vi "CoMP-S Mechanism - AISAS Motor Controller - MK.vi"(8 "Steps/sec (3-365)":dbl=15.0, 9 "Steps":dbl=10.0, 10 "Motor Direction":T1=enum."Rotation Counter Clockwise", 11 "Motor":T2=enum."Rotation") -> (0 "Read Buffer Out":string="\n", 1 "Bytes Read":u32=1, 2 "Estimated time [sec]":dbl=0.9876666666666667, 3 "sec":ext=0.62100000000000000003)   [LabVIEW 2014]
doc: "Rotation Definition when Looking at the Sun. CCW, Right is CW, Optimum speed is 10 steps/s\n\nDiffuser opens with 1200 total steps, optimum speed is 10 steps/s\n\nObjective Lens\n\n\nvelocity = 730,88/steps.p.sec"
uses:
  AISAS Mechanism Action Type Def.ctl
  AISAS Mechanism Action Direction Type Def.ctl
panel:
  out "ERROR":bool
  in  "bytes  to read":i32=1
  # "Time [sec]"
  # "k"
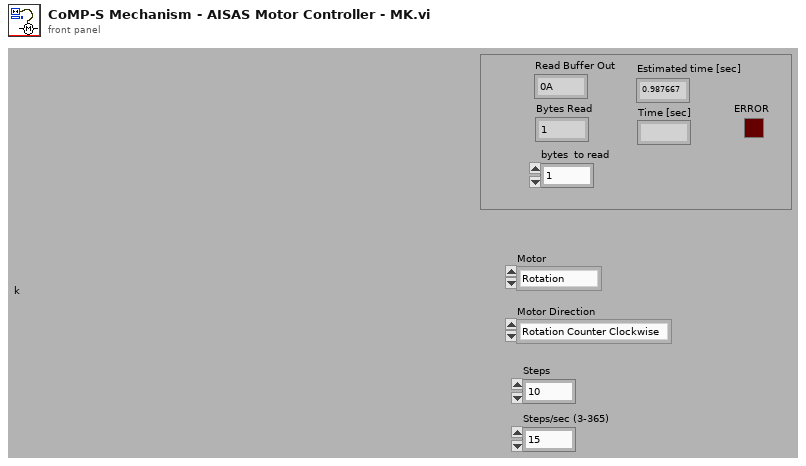
[diagram p1: front panel]
types:
  T1 = typedef "AISAS Mechanism Action Direction Type Def.ctl" = enum16{"Diffuser Closed", "Diffuser Open", "Objective Lens Away", "Objective Lens Closer", "Rotation Counter Clockwise", "Rotation Clockwise"}
  T2 = typedef "AISAS Mechanism Action Type Def.ctl" = enum16{"Diffuser", "Objective Lens", "Rotation"}
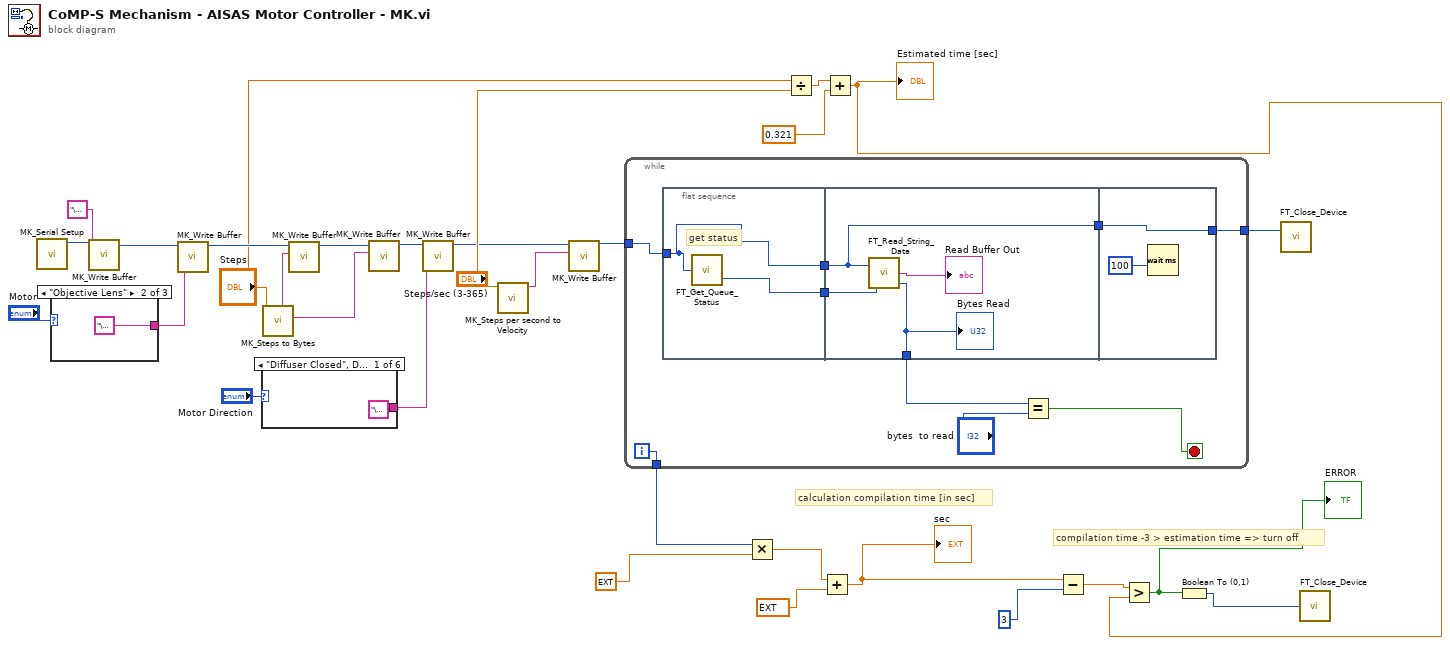
[diagram p0: block diagram]
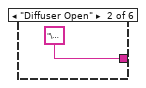
[diagram p2: hidden frame]
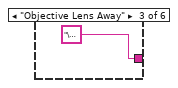
[diagram p3: hidden frame]
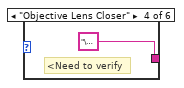
[diagram p4: hidden frame]
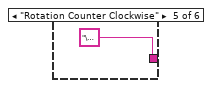
[diagram p5: hidden frame]
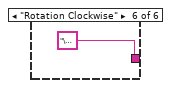
[diagram p6: hidden frame]
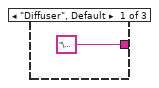
[diagram p7: hidden frame]
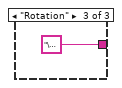
[diagram p8: hidden frame]
diagram:
  # "compilation time -3 > estimation time => turn off"
  # "calculation compilation time [in sec]"
  n1 = call "MK_Serial Setup.vi"() -> ("Handle"=w17:u32)  [unwired: 11 in]
  n2 = case shown="\"Objective Lens\"" "Motor" {
    tunnel: ["\u0003" "\u0004" "\u0002"] -> w14
    frame "Diffuser", Default {
    }
    frame "Objective Lens" {
    }
    frame "Rotation" {
    }
  }
  n3 = call "MK_Write Buffer.vi"("Buffer"="\u0001", "Handle in"=w17) -> ("Handle out"=w13:u32)  [unwired: 9 in]
  n4 = call "MK_Write Buffer.vi"("Buffer"=w14, "Handle in"=w13) -> ("Handle out"=w9:u32)  [unwired: 9 in]
  n5 = case shown="\"Diffuser Closed\", Default" "Motor Direction" {
    tunnel: ["\u0000" "\u0001" "\u0000" "\u0001" "\u0001" "\u0000"] -> w6
    frame "Diffuser Closed", Default {
    }
    frame "Diffuser Open" {
    }
    frame "Objective Lens Away" {
    }
    frame "Objective Lens Closer" {
      # "<Need to verify"
    }
    frame "Rotation Counter Clockwise" {
    }
    frame "Rotation Clockwise" {
    }
  }
  n6 = call "MK_Steps to Bytes.vi"("Steps"="Steps") -> ("Hi Byte"=w10:string, "Lo Byte"=w12:string)  [unwired: 9 in]
  n7 = call "MK_Write Buffer.vi"("Buffer"=w12, "Handle in"=w9) -> ("Handle out"=w11:u32)  [unwired: 9 in]
  n8 = call "MK_Write Buffer.vi"("Buffer"=w10, "Handle in"=w11) -> ("Handle out"=w5:u32)  [unwired: 9 in]
  n9 = call "MK_Write Buffer.vi"("Buffer"=w6, "Handle in"=w5) -> ("Handle out"=w3:u32)  [unwired: 9 in]
  n10 = call "MK_Steps per second to Velocity.vi"("Steps/sec (3-365)"="Steps/sec (3-365)") -> ("Velocity"=w2:string)  [unwired: 10 in]
  n11 = call "MK_Write Buffer.vi"("Buffer"=w2, "Handle in"=w3) -> ("Handle out"=w1:u32)  [unwired: 9 in]
  n12 = while {
    tunnel: w1 -> [w48]
    tunnel: [w42] -> w28
    tunnel: [w40] -> w30
    i -> [w42]
    stop <- w43 stop-if-true
    n13 = flat-sequence {
      tunnel: w48 -> [w49]
      tunnel: [w50] -> w47
      tunnel: [w49] -> w46
      tunnel: w47 -> [w54]
      tunnel: w46 -> [w51]
      tunnel: [w52] -> w44
      tunnel: [w51] -> w41
      tunnel: w41 -> [w55]
      tunnel: [w55] -> w40
      frame #0 {
        # "get status"
        n14 = call "FT_Get_Queue_Status.vi"("Handle"=w49) -> ("Bytes Waiting"=w50:u32)  [unwired: 1 out]
      }
      frame #1 {
        n15 = call "FT_Read_String_Data.vi"("Handle"=w51, "Bytes To Read"=w54) -> ("Read Data"=→"Read Buffer Out":string, "Bytes Read"=w52:u32)  [unwired: 1 out]
        "Bytes Read" <- w52
      }
      frame #2 {
        n16 = Wait (ms)(milliseconds to wait=u32 100) -> ()  [unwired: 1 out]
      }
    }
    n17 = Equal?(x=w44, y="bytes  to read") -> (x = y?=w43:bool)
  }
  n18 = Multiply(x=w28, y=ext 0.1) -> (x*y=w26:ext)
  n19 = Divide(x="Steps", y="Steps/sec (3-365)") -> (x/y=w25:dbl)
  n20 = Add(x=w26, y=ext 0.32099999999999999999) -> (x+y=w23:ext)
  "sec" <- w23
  n21 = Add(x=w25, y=0.321) -> (x+y=w20:dbl)
  "Estimated time [sec]" <- w20
  n22 = Subtract(x=w23, y=3) -> (x-y=w21:ext)
  n23 = Greater?(x=w21, y=w20) -> (0:w18:bool)
  "ERROR" <- w18
  n24 = Boolean To (0,1)(Boolean=w18) -> (0, 1=w19:i16)
  n25 = call "FT_Close_Device.vi"("Handle"=w30) -> ()  [unwired: 1 out]
  n26 = call "FT_Close_Device.vi"("Handle"=w19) -> ()  [unwired: 1 out]
